vi "GetMenuItems.vi"(8 "error in (no error)":errorcluster, 11 "MenuCol in":refnum<class "MenuCol.lvclass">) -> (0 "error out":errorcluster, 1 "MenuTags":string[](array[string]), 2 "MenuLabels":string[](array[string]), 3 "MenuCol out":refnum<class "MenuCol.lvclass">)   [LabVIEW 2013, in "MenuCol.lvclass"]
uses:
  MenuCol.lvclass
  MenuCol.lvclass/MenuCol.ctl
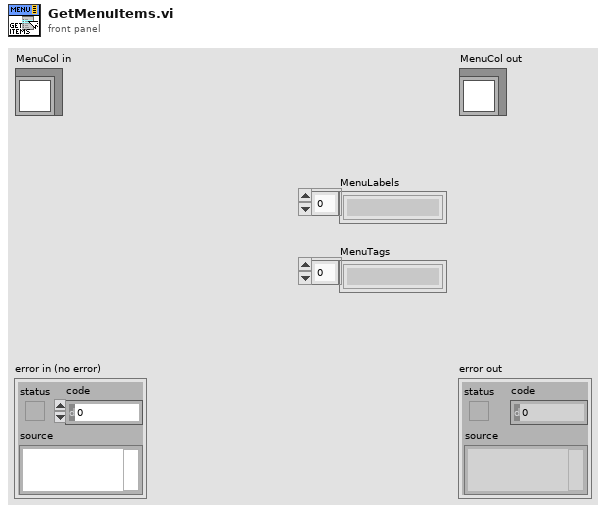
[diagram p1: front panel]
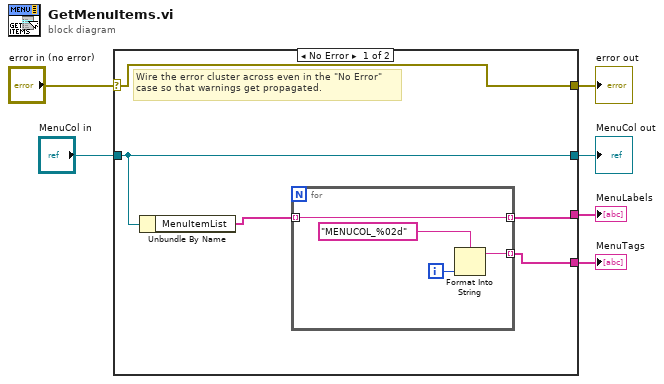
[diagram p0: block diagram]
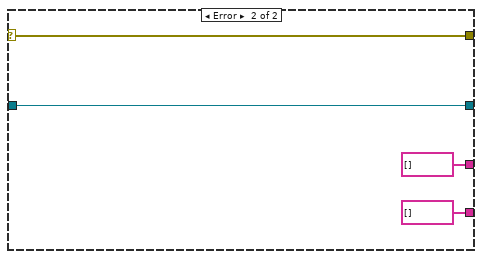
[diagram p2: hidden frame]
diagram:
  n1 = case shown="No Error" "error in (no error)" {
    selector: "error in (no error)" -> [w11 w19]
    tunnel: [w11 w19] -> w5
    tunnel: [w10 w18] -> w3
    tunnel: "MenuCol in" -> [w10 w18]
    tunnel: [w7 string[] []] -> w1
    tunnel: [w8 string[] []] -> w2
    frame No Error {
      # "Wire the error cluster across even in the \"No Error\"\ncase so that warnings get propagated."
      n2 = Unbundle By Name(w10) -> ("MenuItemList"=w9:string[])
      n3 = for {
        tunnel: w9 -> [w15] mode=indexing
        tunnel: [w15] -> w8 mode=indexing
        tunnel: [w13] -> w7 mode=indexing
        i -> [w14]
        n4 = Format Into String(format string="MENUCOL_%02d", w14) -> (resulting string=w13:string)  [unwired: 2 in, 1 out]
      }
    }
    frame Error {
    }
  }
  "error out" <- w5
  "MenuCol out" <- w3
  "MenuLabels" <- w2
  "MenuTags" <- w1
